vi "MALT Get Several.vi"(8 "error in":errorcluster, 9 "Port":i32, 10 "Address":i32, 11 "MALT CardType":T1=enum."MALT132") -> (0 "error out":errorcluster, 3 "Status Map":u8[](array[numeric]) format="%02x")   [LabVIEW 2018]
uses:
  Types/MALT CardTypes.ctl
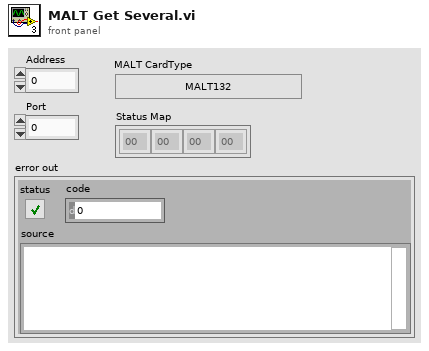
[diagram p1: front panel]
types:
  T1 = typedef "MALT CardTypes.ctl" = enum32{"-", "YAV90832", "YAV904X8", "MALT132", "YAV91616", "YAV90PIN", "YAV90096", "YAV90HVT", "YAV90CLR", "YAV90128", "YAV90PNE", "YAVCANCON", "YAV91775", "YAV90XXX", "YAV90MMU", "H730050", "H710060", "H710061", "YAV90304", "MMI", "YAV90060", "MALT160T", "YAV90059", "Not Defined"}
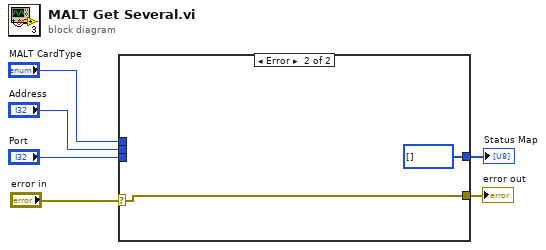
[diagram p0: block diagram]
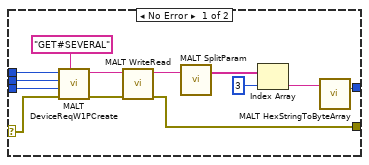
[diagram p2: hidden frame]
diagram:
  n1 = case shown="Error" "error in" {
    selector: "error in" -> [w7 w20]
    tunnel: [w18 w20] -> w6
    tunnel: "Port" -> [w14 _]
    tunnel: "Address" -> [w13 _]
    tunnel: "MALT CardType" -> [w10 _]
    tunnel: [w8 u8[] [] ("Bytes out")] -> w2
    frame No Error {
      n2 = call "MALT DeviceReqW1PCreate.vi"("Cmd"="GET#SEVERAL" ("cmd"), "error in"=w7, "Param1"=w14, "Address"=w13, "CardType"=w10) -> ("error out"=w12:errorcluster, "Request"=w15:string)  [unwired: 5 in]
      n3 = call "MALT WriteRead.vi"("error in"=w12, "Request"=w15) -> ("error out"=w18:errorcluster, "Response"=w19:string)  [unwired: 8 in]
      n4 = call "MALT SplitParam.vi"("Line"=w19) -> ("Items"=w17:string[])  [unwired: 2 in]
      n5 = Index Array(array=w17, index=3) -> (element=w9:string)
      n6 = call "MALT HexStringToByteArray.vi"("String in"=w9) -> ("Bytes out"=w8:u8[])  [unwired: 2 in]
    }
    frame Error {
    }
  }
  "error out" <- w6
  "Status Map" <- w2
